vi "UART 8N1 Command and Response.vi"(6 "Text to Send":string, 7 "Active Dut":T1, 8 "Response Size (char)":u32, 9 "Response Timeout (ms)":i32, 10 "Error In":errorcluster, 11 "FPGA VI Reference In":refnum<k20>) -> (0 "Received Text":string, 1 "Timeout Flag":bool, 2 "Error Out":errorcluster, 3 "FPGA VI Reference Out":refnum<k20>, 5 "Elements Remaining":u32)   [LabVIEW 2018]
uses:
  Resources_Test/UART/ControlTestSlot.ctl
  <vilib>/Utility/error.llb/Error Cluster From Error Code.vi
  <vilib>/rvi/errors/niLvFpgaAdjustHostInterfaceError.vi
  <vilib>/rvi/interface/nirviMethod/nirviMethod.xnode
  Program Files (x86)/National Instruments/LabVIEW 2018/instr.lib/niVST/FPGA/Templates/FPGA Bitfiles/niVSTFPGA_UART.lvbitx
  <vilib>/rvi/errors/niLvFpgaMergeErrorWithErrorCode.vi
  <vilib>/FPGAPlugInAG/PXIe-5840/niLvFpga_WriteFifo_PXIe-5840.vi
  <vilib>/FPGAPlugInAG/PXIe-5840/niLvFpga_ReadFifo_PXIe-5840.vi
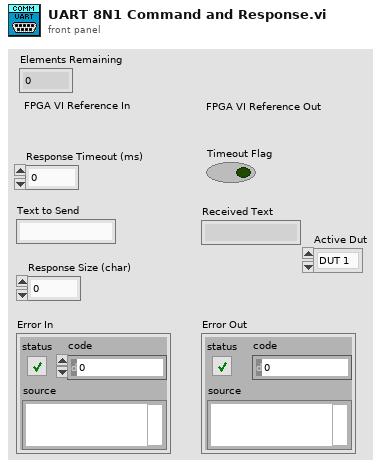
[diagram p1: front panel]
types:
  T1 = typedef "ControlTestSlot.ctl" = enum16{"DUT 1", "DUT 2"}
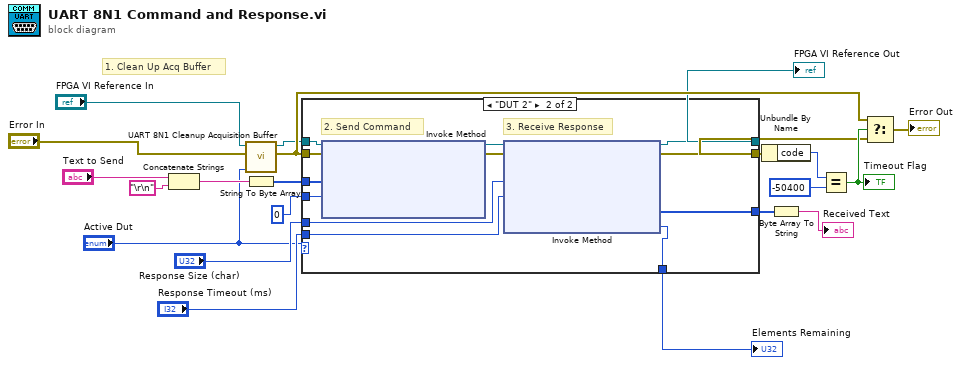
[diagram p0: block diagram]
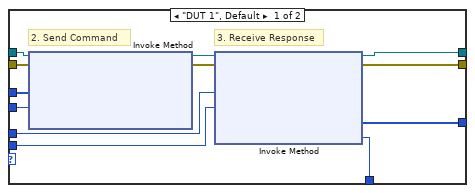
[diagram p2: hidden frame]
diagram:
  # "1. Clean Up Acq Buffer"
  n1 = Concatenate Strings("Text to Send", "\r\n") -> (w16:string)
  n2 = call "UART 8N1 Cleanup Acquisition Buffer.vi"("Active Dut"="Active Dut", "Error In"="Error In", "FPGA VI Reference In"="FPGA VI Reference In") -> ("Error Out"=w7:errorcluster, "FPGA VI Reference Out"=w3:refnum<k20>)  [unwired: 6 in, 1 out]
  n3 = String To Byte Array(string=w16) -> (unsigned byte array=w12:u8[])
  n4 = case shown="\"DUT 2\"" "Active Dut" {
    tunnel: w7 -> [w32 w45]
    tunnel: w12 -> [w31 w44]
    tunnel: 0 ("Timeout (ms)") -> [w30 w43]
    tunnel: [w27 w39] -> w5
    tunnel: [w26 w38] -> w6
    tunnel: w3 -> [w33 w42]
    tunnel: "Response Size (char)" -> [w25 w37]
    tunnel: "Response Timeout (ms)" -> [w24 w36]
    tunnel: [w23 w35] -> w8
    tunnel: [w22 w34] -> w2
    frame "DUT 1", Default {
      # "3. Receive Response"
      # "2. Send Command"
      n5 = xnode "Invoke Method"("FPGA VI Reference In"=w33, "error in"=w32, "Data"=w31, "Timeout (ms)"=w30) -> ("FPGA VI Reference Out"=w29:refnum<k20>, "error out"=w28:errorcluster)  [unwired: 1 out]
      n6 = xnode "Invoke Method"("FPGA VI Reference In"=w29, "error in"=w28, "Number of Elements"=w25, "Timeout (ms)"=w24) -> ("FPGA VI Reference Out"=w27:refnum<k20>, "error out"=w26:errorcluster, "Data"=w23:u32[], "Elements Remaining"=w22:u32)
    }
    frame "DUT 2" {
      # "3. Receive Response"
      # "2. Send Command"
      n7 = xnode "Invoke Method"("FPGA VI Reference In"=w42, "error in"=w45, "Data"=w44, "Timeout (ms)"=w43) -> ("FPGA VI Reference Out"=w41:refnum<k20>, "error out"=w40:errorcluster)  [unwired: 1 out]
      n8 = xnode "Invoke Method"("FPGA VI Reference In"=w41, "error in"=w40, "Number of Elements"=w37, "Timeout (ms)"=w36) -> ("FPGA VI Reference Out"=w39:refnum<k20>, "error out"=w38:errorcluster, "Data"=w35:u32[], "Elements Remaining"=w34:u32)
    }
  }
  "FPGA VI Reference Out" <- w5
  "Elements Remaining" <- w2
  n9 = Unbundle By Name(w6) -> ("code"=w19:i32)
  n10 = Byte Array To String(unsigned byte array=w8) -> (string=→"Received Text":string)
  n11 = Equal?(x=w19, y=-50400) -> (x = y?=w17:bool)
  "Timeout Flag" <- w17
  n12 = Select(t=w7, s=w17, f=w6) -> (s? t:f=→"Error Out":errorcluster)
